vi "Format Gas Params.vi"() -> ()   [LabVIEW 2014]
panel:
  out "error out":errorcluster
  in  "error in":errorcluster
  out "Result":string="Temperature: 1.000000\r Pressure: 2.000000\r Humidity: 3.000000\r Volume: 4.000000 \r Density: 5.000000"
  in  "Density":dbl=5.0
  in  "Volume":dbl=4.0
  in  "Humidity":dbl=3.0
  in  "Pressure":dbl=2.0
  in  "Temperature":dbl=1.0
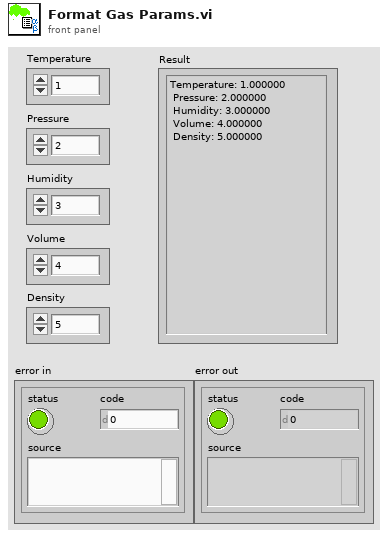
[diagram p1: front panel]
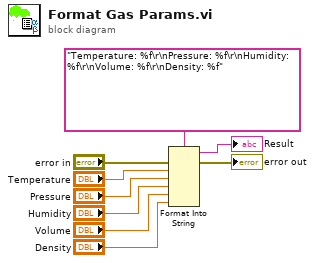
[diagram p0: block diagram]
diagram:
  n1 = Format Into String(format string="Temperature: %f\r\nPressure: %f\r\nHumidity: %f\r\nVolume: %f\r\nDensity: %f", error in="error in", "Temperature", "Pressure", "Humidity", "Volume", "Density") -> (resulting string=→"Result":string, error out=→"error out":errorcluster)  [unwired: 1 in]
